vi "2dinterpolatetest.vi"() -> ()   [LabVIEW 2011]
uses:
  <vilib>/gmath/interp.llb/Interpolate 2D (1d xi,yi).vi
  <vilib>/gmath/NI_Gmath.lvlib
panel:
  in  "yi":dbl[](array[numeric])
  in  "xi":dbl[](array[numeric])
  out "zi":dbl[][](array[numeric])
  in  "Y":dbl[](array[numeric])
  in  "X":dbl[](array[numeric])
  in  "Z":dbl[][](array[numeric])
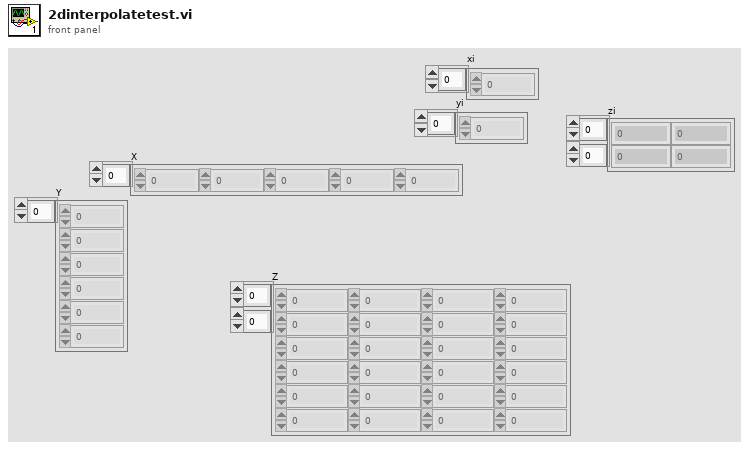
[diagram p1: front panel]
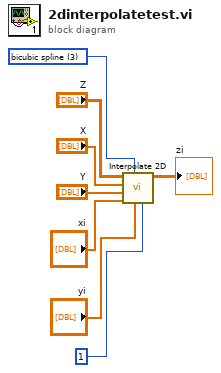
[diagram p0: block diagram]
diagram:
  w8 = 3 items=["nearest", "bilinear", "bicubic", "bicubic spline"] ("method")
  n1 = call-poly <vilib>:"Interpolate 2D.vi"("ntimes"=1, "yi"="yi", "method"=w8, "xi"="xi", "Y"="Y", "X"="X", "Z"="Z") -> ("zi"=→"zi":dbl[][])  [unwired: 1 in, 3 out]
